vi "one_button.vi"(7 "callee":refnum<vi>, 8 "error in (no error)":errorcluster, 11 "configuration":T2={"dialog_text"="", "boolean_text_1"="", "boolean_text_2"="", "boolean_text_3"="", "inner_color"=16711680, "outer_color"=6618880, "wait_s"=nan, "error_status"=FALSE, "error_source"="", "error_details"="", "string []"=[], "custom_entry"=FALSE}) -> (0 "error out":errorcluster, 3 "dialog_selection":T1)   [LabVIEW 2015, in "lv-dialog-interfaces.lvlib"]
uses:
  lv-dialog-interfaces.lvlib
  lv-dialog/api/v1/public/_controls/configuration.ctl
  lv-dialog/api/v1/public/_controls/dialog_selection.ctl
  _controls/dialog_type.ctl
  _controls/hmi_references.ctl
  <vilib>/event_ctls.llb/eventvkey.ctl
  lv-dialog/api/v1/v1.lvlib
panel:
  out "dialog":string
  in  "button_1":bool
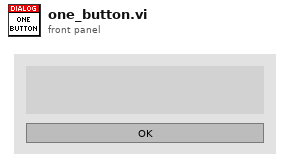
[diagram p1: front panel]
types:
  T1 = typedef "lv-dialog.lvlib/v1.lvlib/dialog_selection.ctl" = enum16{"null", "panel_closed", "button_1", "button_2", "button_3", "cancelled"}
  T2 = typedef "lv-dialog.lvlib/v1.lvlib/configuration.ctl" = cluster{"dialog_text":string, "boolean_text_1":string, "boolean_text_2":string, "boolean_text_3":string, "inner_color":u32, "outer_color":u32, "wait_s":dbl, "error_status":bool, "error_source":string, "error_details":string, "string []":string[], "custom_entry":bool}
  T3 = typedef "lv-dialog-interfaces.lvlib/dialog_type.ctl" = enum16{"null", "one_button", "two_button", "three_button", "confirmation", "busy_wait", "error", "busy_wait_embed", "combo_box", "data_entry_string", "data_entry_numeric"}
  T4 = typedef "lv-dialog-interfaces.lvlib/hmi_references.ctl" = cluster{"vi_reference":refnum<vi>, "caller":refnum<vi>, "dialog":refnum<vi>, "button_1":refnum<vi>, "button_2":refnum<vi>, "button_3":refnum<vi>, "busy":refnum<vi>, "error_glyph":refnum<vi>, "error_source":refnum<vi>, "error_text":refnum<vi>, "combo_box":refnum<vi>}
  T5 = typedef "eventvkey.ctl" = enum16{"ASCII", "Enter", "Return", "Shift", "Ctrl", "Alt", "Cmd", "Opt", "Caps", "NumLock", "Clear", "Break", "Up", "Down", "Left", "Right", "Insert", "Delete", "Home", "End", "PageUp", "PageDown", "Escape", "Help", "Pause", "ScrollLock", "F1", "F2", "F3", "F4", "F5", "F6", "F7", "F8", "F9", "F10", "F11", "F12", "F13", "F14", "F15", "F16", "F17", "F18", "F19", "F20", "F21", "F22", "F23", "F24", "Play", "VolumeUp", "VolumeDown", "Mute", "Two Byte Char"}
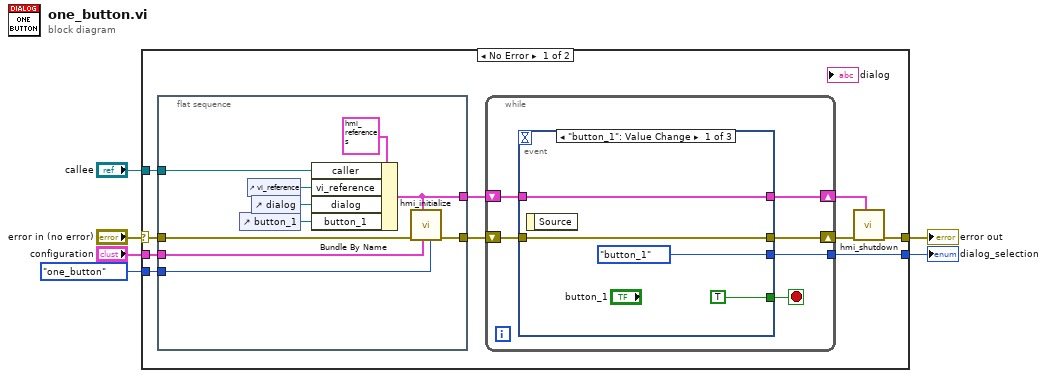
[diagram p0: block diagram]
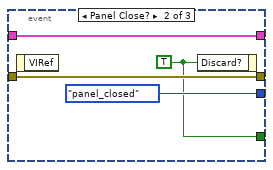
[diagram p2: hidden frame]
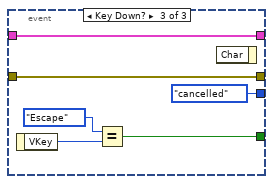
[diagram p3: hidden frame]
diagram:
  n1 = case shown="No Error" "error in (no error)" {
    selector: "error in (no error)" -> [w16 w47]
    tunnel: "configuration" -> [w15 _]
    tunnel: dialog_type."one_button" ("dialog_type") -> [w14 _]
    tunnel: [w12 _] -> w3
    tunnel: "callee" -> [w11 _]
    tunnel: [w9 w47] -> w1
    frame No Error {
      n2 = flat-sequence {
        tunnel: w16 -> [w19]
        tunnel: w15 -> [w22]
        tunnel: w14 -> [w21]
        tunnel: [w20] -> w13
        tunnel: w11 -> [w18]
        tunnel: [w17] -> w8
        frame #0 {
          n3 = control-ref of="button_1"() -> (w24:refnum<vi>)
          n4 = control-ref of="vi_reference"() -> (w26:refnum<vi>)
          n5 = control-ref of="dialog"() -> (w25:refnum<vi>)
          n6 = Bundle By Name(cluster=T4 {"vi_reference"=refnum, "caller"=refnum, "dialog"=refnum, "button_1"=refnum, "button_2"=refnum, "button_3"=refnum, "busy"=refnum, "error_glyph"=refnum, "error_source"=refnum, "error_text"=refnum, "combo_box"=refnum}, "caller"=w18, "vi_reference"=w26, "dialog"=w25, "button_1"=w24) -> (w17:T4)
          n7 = call "hmi_initialize.vi"("dialog_type"=w21, "configuration"=w22, "references"=w17, "error in (no error)"=w19) -> ("error out"=w20:errorcluster)  [unwired: 7 in]
        }
      }
      n8 = while {
        tunnel: [w30] -> w12
        shift-right: [w31] -> w10
        shift-left: w13 -> [w32]
        shift-right: [w28] -> w7
        shift-left: w8 -> [w29]
        stop <- w27 stop-if-true
        n9 = event shown="[0] \"button_1\": Value Change" {
          selector: _ -> [_ _ _]
          dyn-events: _ -> [_ _ _]
          timeout: _ -> [_ _ _]
          tunnel: w32 -> [w36 w40 w41]
          tunnel: [w36 w40 w41] -> w31
          tunnel: [dialog_selection."button_1" ("dialog_selection") dialog_selection."panel_closed" ("dialog_selection") dialog_selection."cancelled" ("dialog_selection")] -> w30
          tunnel: w29 -> [w34 w38 w46]
          tunnel: [w34 w38 w46] -> w28
          tunnel: [TRUE w37 w43] -> w27
          event "button_1": Value Change {
            n10 = event-data() -> ()  [unwired: 1 in, 1 out]
          }
          event Panel Close? {
            w37 = TRUE ("Discard?")
            n11 = event-data() -> ()  [unwired: 1 in, 1 out]
            n12 = event-data("Discard?"=w37) -> ()  [unwired: 1 in, 1 out]
          }
          event Key Down? {
            n13 = event-data() -> ("VKey"=w45:T5)  [unwired: 1 in]
            n14 = Equal?(x=eventvkey."Escape" ("VKey"), y=w45) -> (x = y?=w43:bool)
            n15 = event-data() -> ()  [unwired: 2 in, 1 out]
          }
        }
      }
      n16 = call "hmi_shutdown.vi"("references"=w7, "error in (no error)"=w10) -> ("error out"=w9:errorcluster)  [unwired: 9 in]
    }
    frame Error {
    }
  }
  "error out" <- w1
  "dialog_selection" <- w3
